vi "Open Connection.vi"(2 "error in (no error)":errorcluster) -> (0 "error out":errorcluster, 1 "Database.lvlib:Data Store.lvclass":refnum<class "Data Store.lvclass">)   [LabVIEW 2012, in "Database.lvlib" / "Data Store.lvclass"]
uses:
  Data Store.lvclass
  Data Store.lvclass/Data Store.ctl
  <vilib>/addons/database/Connection.llb/DB Tools Open Connec (String).vi
  <vilib>/addons/database/NI_Database_API.lvlib
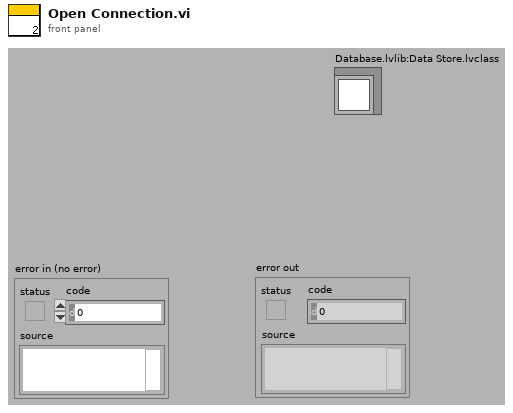
[diagram p1: front panel]
types:
  T1 = typedef "NI_Database_API.lvlib/Conn ObjectReference.ctl" = refnum<k1>
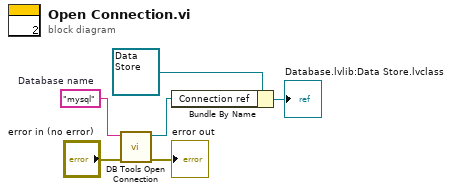
[diagram p0: block diagram]
diagram:
  w1 = "mysql"  # Database name
  n1 = call-poly <vilib>:"DB Tools Open Connection.vi"("error in (no error)"="error in (no error)", "connection information"=w1) -> ("error out"=→"error out":errorcluster, "connection reference"=w4:T1)  [unwired: 6 in]
  n2 = Bundle By Name(cluster=refnum<class "Data Store.lvclass"> refnum ("Database.lvlib:Data Store Connection.lvclass 2"), "Connection ref"=w4) -> (→"Database.lvlib:Data Store.lvclass":refnum<class "Data Store.lvclass">)
